vi "Chute.vi"(11 "Enable  Chute":bool) -> ()   [LabVIEW 2019, in "8085 VI Library.lvlib"]
uses:
  <vilib>/Rock Robotics/WPI/ThirdParty/Phoenix-LabVIEW/Motor Controller/Controls/CTRE_Phoenix_MotorControl_ControlMode.ctl
  <vilib>/Rock Robotics/WPI/Solenoid/WPI_SolenoidValue.ctl
  <vilib>/Rock Robotics/WPI/Solenoid/WPI_SolenoidSetEnum.vi
  8085 VI Library.lvlib
panel:
  in  "Control Mode 7":T1 items=["PercentOutput"=0, "Position"=1, "Velocity"=2, "Current"=3, "Follower"=5, "MotionProfile"=6, "MotionMagic"=7, "MotionProfileArc"=10, "Disabled"=15]
  in  "Control Mode 8":T1 items=["PercentOutput"=0, "Position"=1, "Velocity"=2, "Current"=3, "Follower"=5, "MotionProfile"=6, "MotionMagic"=7, "MotionProfileArc"=10, "Disabled"=15]
  in  "Control Mode 9":T1 items=["PercentOutput"=0, "Position"=1, "Velocity"=2, "Current"=3, "Follower"=5, "MotionProfile"=6, "MotionMagic"=7, "MotionProfileArc"=10, "Disabled"=15]
  in  "Control Mode 6":T1 items=["PercentOutput"=0, "Position"=1, "Velocity"=2, "Current"=3, "Follower"=5, "MotionProfile"=6, "MotionMagic"=7, "MotionProfileArc"=10, "Disabled"=15]
  in  "Control Mode 5":T1 items=["PercentOutput"=0, "Position"=1, "Velocity"=2, "Current"=3, "Follower"=5, "MotionProfile"=6, "MotionMagic"=7, "MotionProfileArc"=10, "Disabled"=15]
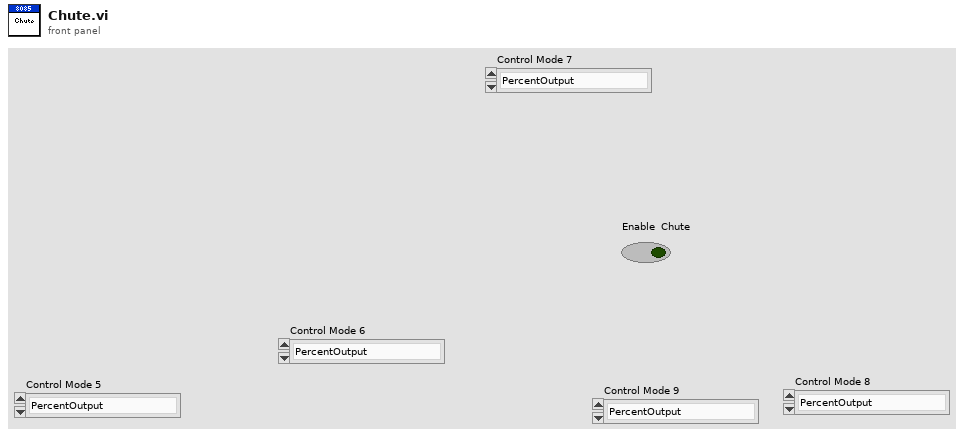
[diagram p1: front panel]
types:
  T1 = typedef "CTRE_Phoenix_MotorControl_ControlMode.ctl" = u16
  T2 = typedef "WPI_SolenoidDevRef.ctl" = cluster{"DevStatus":errorcluster, "Pneumatics Control Module":u8, "Forward Solenoid Channel":T3, "Reverse Solenoid Channel":T3}
  T3 = typedef "WPI_SolenoidChannel.ctl" = enum8{"Solenoid 0", "Solenoid 1", "Solenoid 2", "Solenoid 3", "Solenoid 4", "Solenoid 5", "Solenoid 6", "Solenoid 7", "Invalid"}
  T4 = typedef "WPI_SolenoidValue.ctl" = enum16{"Off", "On", "Forward", "Reverse"}
  T5 = typedef "WPI_MotorControlDeviceRef.ctl" = cluster{"DeviceStatus":errorcluster, "Type":T6, "PWM":cluster{"PWM Channel":T7, "DeadBand":T8}, "CAN":cluster{"Device Number":u8, "SetOutput VI Ref":variant, "GetOutput VI Ref":variant, "Enable VI Ref":variant, "Disable VI Ref":variant, "Data":variant}, "Invert":bool, "DIO PWM":cluster{"PWM \"Enable\" Channel":T7, "DIOChannel":T9, "PWM Rate":dbl}}
  T6 = typedef "WPI_MotorControlType.ctl" = enum16{"PWM", "CAN", "DIO PWM"}
  T7 = typedef "FPGA_DIOPWMChannel.ctl" = enum8{"PWM 0", "PWM 1", "PWM 2", "PWM 3", "PWM 4", "PWM 5", "PWM 6", "PWM 7", "PWM 8", "PWM 9", "PWM MXP 0", "PWM MXP 1", "PWM MXP 2", "PWM MXP 3", "PWM MXP 4", "PWM MXP 5", "PWM MXP 6", "PWM MXP 7", "PWM MXP 8", "PWM MXP 9", "Invalid"}
  T8 = typedef "WPI_PWMDeadband.ctl" = cluster{"Name":string, "maxPositivePwm":i32, "minPositivePwm":i32, "centerPwm":i32, "maxNegativePwm":i32, "minNegativePwm":i32, "angularRange":u16}
  T9 = typedef "FPGA_DIOChannel.ctl" = enum8{"DIO 0", "DIO 1", "DIO 2", "DIO 3", "DIO 4", "DIO 5", "DIO 6", "DIO 7", "DIO 8", "DIO 9", "DIO MXP 0", "DIO MXP 1", "DIO MXP 2", "DIO MXP 3", "DIO MXP 4", "DIO MXP 5", "DIO MXP 6", "DIO MXP 7", "DIO MXP 8", "DIO MXP 9", "DIO MXP 10", "DIO MXP 11", "DIO MXP 12", "DIO MXP 13", "DIO MXP 14", "DIO MXP 15", "SPI Port CS1", "SPI Port CS2", "SPI Port CS3", "SPI Port MISO", "SPI Port MOSI", "Invalid"}
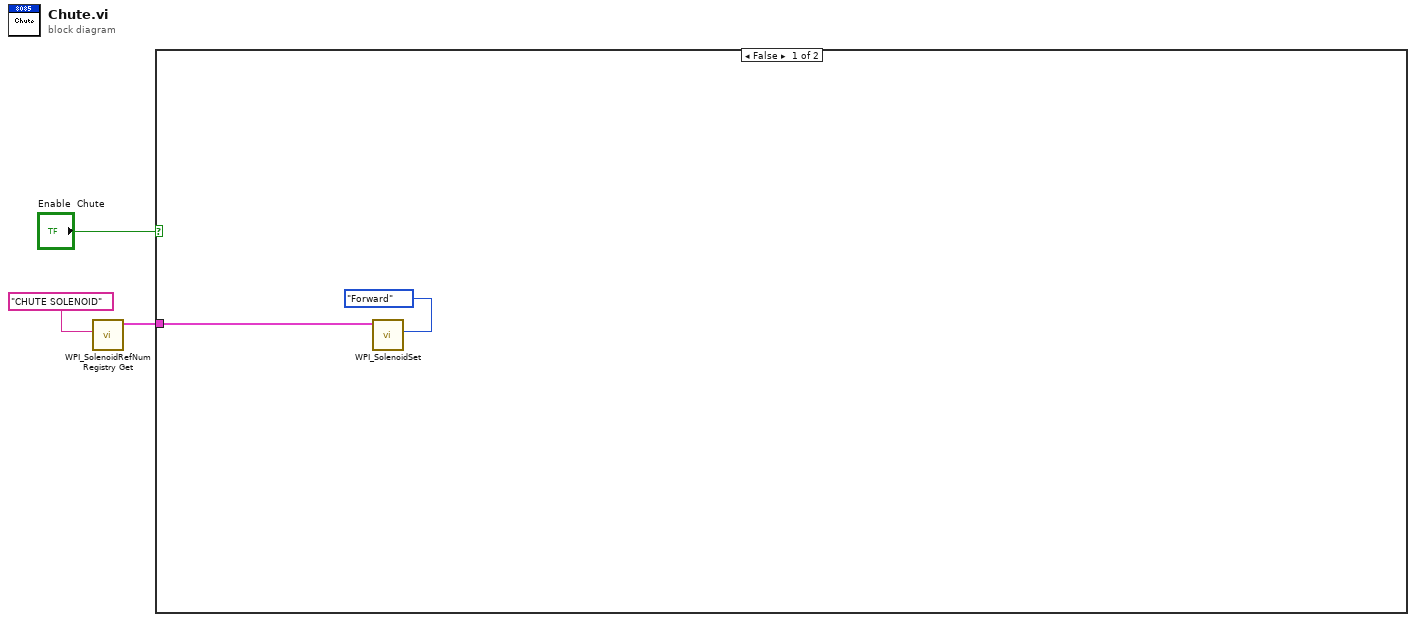
[diagram p0: block diagram]
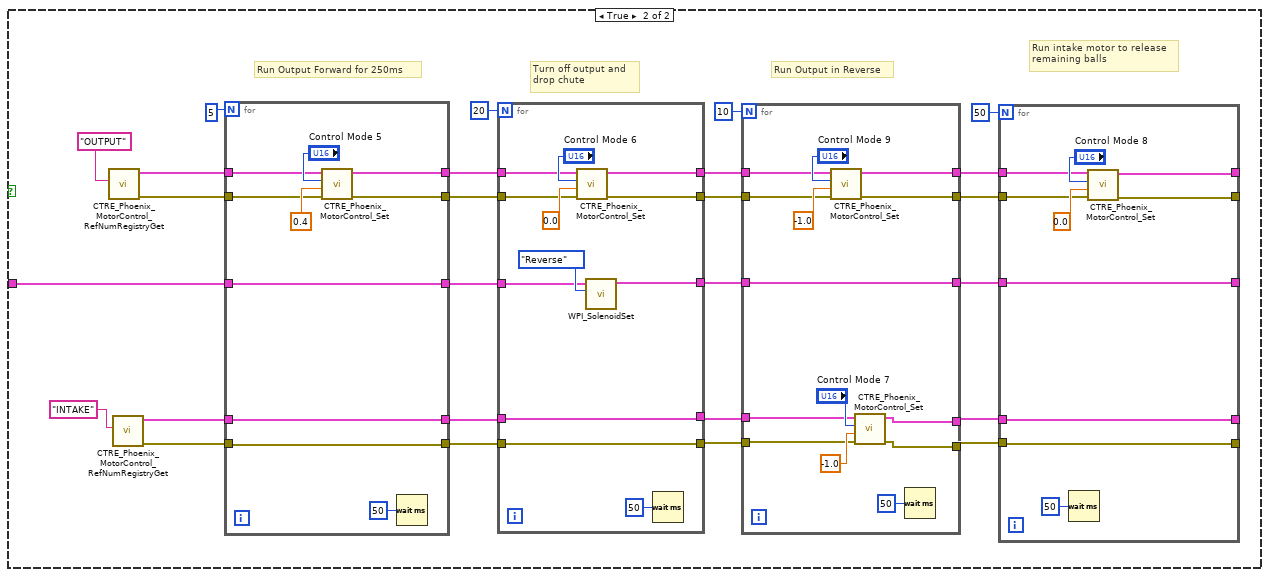
[diagram p2: hidden frame]
diagram:
  n1 = call <vilib>:"WPI_SolenoidRefNum Registry Get.vi"("refnum name"="CHUTE SOLENOID") -> ("SolenoidDevRef"=w1:T2)  [unwired: 9 in, 1 out]
  n2 = case shown="False" "Enable  Chute" {
    tunnel: w1 -> [w4 w6]
    frame False {
      n3 = call-poly <vilib>:"WPI_SolenoidSet.vi"("Value"=WPI_SolenoidValue."Forward", "SolenoidDevRef"=w4) -> ()  [unwired: 8 in, 2 out]
    }
    frame True {
      # "Run intake motor to release\nremaining balls"
      # "Run Output in Reverse"
      # "Turn off output and\ndrop chute"
      # "Run Output Forward for 250ms"
      n4 = call <vilib>:"CTRE_Phoenix_MotorControl_RefNumRegistryGet.vi"("refnum name"="OUTPUT") -> ("error out"=w21:errorcluster, "PhoenixMotorControlDevRef"=w22:T5)  [unwired: 9 in]
      n5 = call <vilib>:"CTRE_Phoenix_MotorControl_RefNumRegistryGet.vi"("refnum name"="INTAKE") -> ("error out"=w27:errorcluster, "PhoenixMotorControlDevRef"=w29:T5)  [unwired: 9 in]
      n6 = for {
        N: 5 -> [_]
        tunnel: w29 -> [w68]
        tunnel: [w69] -> w25
        tunnel: w27 -> [w69]
        tunnel: w22 -> [w74]
        tunnel: w21 -> [w73]
        tunnel: [w72] -> w20
        tunnel: [w71] -> w19
        tunnel: w6 -> [w70]
        tunnel: [w70] -> w18
        tunnel: [w68] -> w8
        n7 = call <vilib>:"CTRE_Phoenix_MotorControl_Set.vi"("error in (no error)"=w73, "Output"=0.4, "Control Mode"="Control Mode 5", "PhoenixMotorControlDevRef"=w74) -> ("error out"=w71:errorcluster, "PhoenixMotorControlDevRef"=w72:T5)  [unwired: 6 in]
        n8 = Wait (ms)(milliseconds to wait=u32 50) -> ()  [unwired: 1 out]
      }
      n9 = for {
        N: 20 -> [_]
        tunnel: w8 -> [w66]
        tunnel: [w66] -> w28
        tunnel: [w65] -> w26
        tunnel: w25 -> [w65]
        tunnel: w20 -> [w62]
        tunnel: w19 -> [w61]
        tunnel: w18 -> [w59]
        tunnel: [w58] -> w17
        tunnel: [w57] -> w16
        tunnel: [w56] -> w15
        n10 = call <vilib>:"CTRE_Phoenix_MotorControl_Set.vi"("error in (no error)"=w61, "Output"=0.0, "Control Mode"="Control Mode 6", "PhoenixMotorControlDevRef"=w62) -> ("error out"=w56:errorcluster, "PhoenixMotorControlDevRef"=w57:T5)  [unwired: 6 in]
        n11 = call-poly <vilib>:"WPI_SolenoidSet.vi"("Value"=WPI_SolenoidValue."Reverse", "SolenoidDevRef"=w59) -> ("SolenoidDevRef"=w58:T2)  [unwired: 8 in, 1 out]
        n12 = Wait (ms)(milliseconds to wait=u32 50) -> ()  [unwired: 1 out]
      }
      n13 = for {
        N: 10 -> [_]
        tunnel: w28 -> [w45]
        tunnel: w26 -> [w44]
        tunnel: [w43] -> w13
        tunnel: [w42] -> w12
        tunnel: w17 -> [w50]
        tunnel: w16 -> [w52]
        tunnel: w15 -> [w51]
        tunnel: [w50] -> w11
        tunnel: [w49] -> w10
        tunnel: [w48] -> w9
        n14 = call <vilib>:"CTRE_Phoenix_MotorControl_Set.vi"("error in (no error)"=w51, "Output"=-1.0, "Control Mode"="Control Mode 9", "PhoenixMotorControlDevRef"=w52) -> ("error out"=w48:errorcluster, "PhoenixMotorControlDevRef"=w49:T5)  [unwired: 6 in]
        n15 = call <vilib>:"CTRE_Phoenix_MotorControl_Set.vi"("error in (no error)"=w44, "Output"=-1.0, "Control Mode"="Control Mode 7", "PhoenixMotorControlDevRef"=w45) -> ("error out"=w42:errorcluster, "PhoenixMotorControlDevRef"=w43:T5)  [unwired: 6 in]
        n16 = Wait (ms)(milliseconds to wait=u32 50) -> ()  [unwired: 1 out]
      }
      n17 = for {
        N: 50 -> [_]
        tunnel: w13 -> [w32]
        tunnel: w12 -> [w33]
        tunnel: w11 -> [w40]
        tunnel: [w40] -> _
        tunnel: w10 -> [w37]
        tunnel: w9 -> [w36]
        tunnel: [w35] -> _
        tunnel: [w34] -> _
        tunnel: [w32] -> _
        tunnel: [w33] -> _
        n18 = Wait (ms)(milliseconds to wait=u32 50) -> ()  [unwired: 1 out]
        n19 = call <vilib>:"CTRE_Phoenix_MotorControl_Set.vi"("error in (no error)"=w36, "Output"=0.0, "Control Mode"="Control Mode 8", "PhoenixMotorControlDevRef"=w37) -> ("error out"=w34:errorcluster, "PhoenixMotorControlDevRef"=w35:T5)  [unwired: 6 in]
      }
    }
  }
